vi "Cluster.vi"(9 "Cluster":T1={"Numeric"=0.0, "String"="", "Cluster"={"Numeric"=0.0, "Cluster"={"Boolean"=FALSE, "Ring"=11}}} {"Cluster"."Cluster"."Ring" items=["aaaa"=11, "bbbb"=22, "cccc"=33]}, 10 "String":string, 11 "Numeric":dbl) -> (3 "Cluster 2":T1={"Numeric"=0.0, "String"="", "Cluster"={"Numeric"=0.0, "Cluster"={"Boolean"=FALSE, "Ring"=11}}} {"Cluster"."Cluster"."Ring" items=["aaaa"=11, "bbbb"=22, "cccc"=33]})   [LabVIEW 2013]
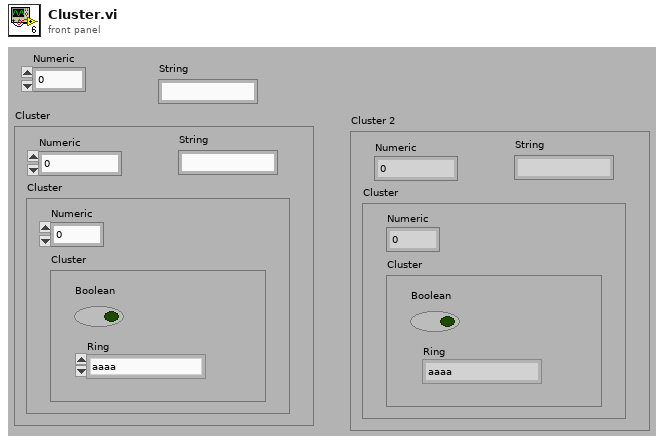
[diagram p1: front panel]
types:
  T1 = cluster{"Numeric":dbl, "String":string, "Cluster":cluster{"Numeric":dbl, "Cluster":cluster{"Boolean":bool, "Ring":i16}}}
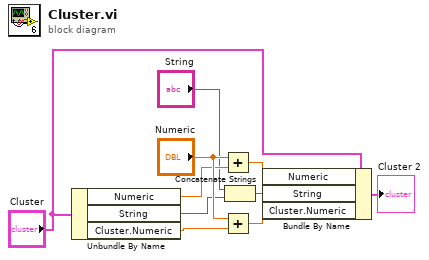
[diagram p0: block diagram]
diagram:
  n1 = Unbundle By Name("Cluster") -> ("Numeric"=w9:dbl, "String"=w6:string, "Cluster.Numeric"=w8:dbl)
  n2 = Add(x="Numeric", y=w9) -> (x+y=w3:dbl)
  n3 = Add(x="Numeric", y=w8) -> (x+y=w1:dbl)
  n4 = Concatenate Strings("String", w6) -> (w2:string)
  n5 = Bundle By Name(cluster="Cluster", "Numeric"=w3, "String"=w2, "Cluster.Numeric"=w1) -> (→"Cluster 2":T1)
